vi "2.2.vi"() -> ()   [LabVIEW 2020]
panel:
  out "element":dbl
  in  "Array":dbl[](array[numeric])
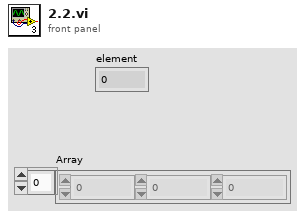
[diagram p1: front panel]
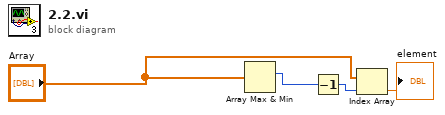
[diagram p0: block diagram]
diagram:
  n1 = Array Max & Min(array="Array") -> (max index (indices)=w2:i32)  [unwired: 3 out]
  n2 = Decrement(x=w2) -> (x-1=w4:i32)
  n3 = Index Array(array="Array", index=w4) -> (element=→"element":dbl)
